vi "对话框.vi"() -> (2 "数值 4":dbl, 3 "数值 3":dbl)   [LabVIEW 2018]
panel:
  in  "取消":bool
  in  "确定":bool
  in  "数值 2":dbl
  in  "数值":dbl
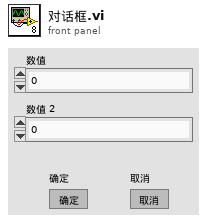
[diagram p1: front panel]
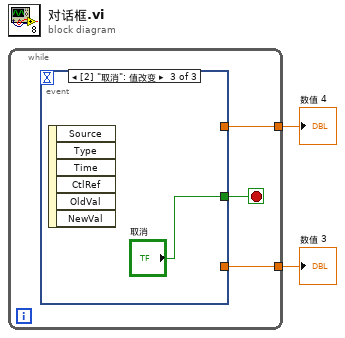
[diagram p0: block diagram]
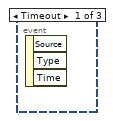
[diagram p2: hidden frame]
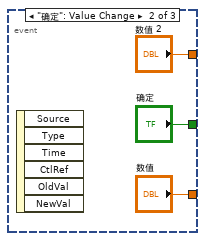
[diagram p3: hidden frame]
diagram:
  n1 = while {
    tunnel: [w5] -> w2
    tunnel: [w4] -> w1
    stop <- w3 stop-if-true
    n2 = event shown="[2] \"取消\": 值改变" {
      selector: _ -> [_ _ _]
      dyn-events: _ -> [_ _ _]
      timeout: _ -> [_ _ _]
      tunnel: [_ "数值" _] -> w5
      tunnel: [_ "数值 2" _] -> w4
      tunnel: [_ "确定" "取消"] -> w3
      event Timeout {
        n3 = event-data() -> ()  [unwired: 1 in, 3 out]
      }
      event "确定": Value Change {
        n4 = event-data() -> ()  [unwired: 1 in, 6 out]
      }
      event "取消": Value Change {
        n5 = event-data() -> ()  [unwired: 1 in, 6 out]
      }
    }
  }
  "数值 3" <- w2
  "数值 4" <- w1
